vi "SyncTag_2.0 Test v2.vi"() -> ()   [LabVIEW 2017]
uses:
  <vilib>/Utility/error.llb/DialogType.ctl
  <vilib>/DAQmx/write.llb/DAQmx Write (Digital Wfm 1Chan NSamp).vi
  <vilib>/Waveform/DWDTOps.llb/DWDT Digital Size.vi
  <vilib>/DAQmx/create/channels.llb/DAQmx Create Channel (DO-Digital Output).vi
  <vilib>/DAQmx/configure/timing.llb/DAQmx Timing (Sample Clock).vi
  <vilib>/Waveform/DWDTOps.llb/DWDT Uncompress Digital.vi
  <vilib>/DAQmx/miscellaneous.llb/DAQmx Fill In Error Info.vi
  <resource>/objmgr/daqmx.rc
panel:
  in  "Sync Tagging":T1(tab)
  out "Minimum tagging period (pws)":u32=87
  out "Total tag data length (pws)":i32=86
  in  "TaggingPeriod (pws)":u32=155
  out "Tag data does NOT fit in period!!!":bool
  in  "Calculate recommended tag settings":bool
  in  "Validate tag settings":bool
  in  "Line(s)":tag="Dev1/port0/line0:7"
  out "Actual Sample Rate":dbl=1000.0 format="%0.2f"
  in  "Sample Clock Source":tag="PFI0"
  in  "Sample Rate":dbl=1000.0
  in  "TagMarkerDuration (pws)":i32=10
  out "digital waveform":digitalwaveform(graph)
  out "Tag num":u32=1
  in  "Min extra tag separation (pws)":u32=1
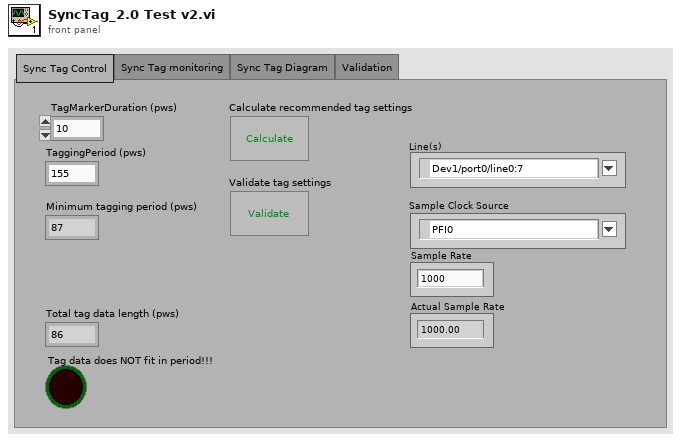
[diagram p1: front panel]
types:
  T1 = enum32{"Sync Tag Control", "Sync Tag monitoring", "Sync Tag Diagram", "Validation"}
  T2 = typedef "DialogType.ctl" = u16
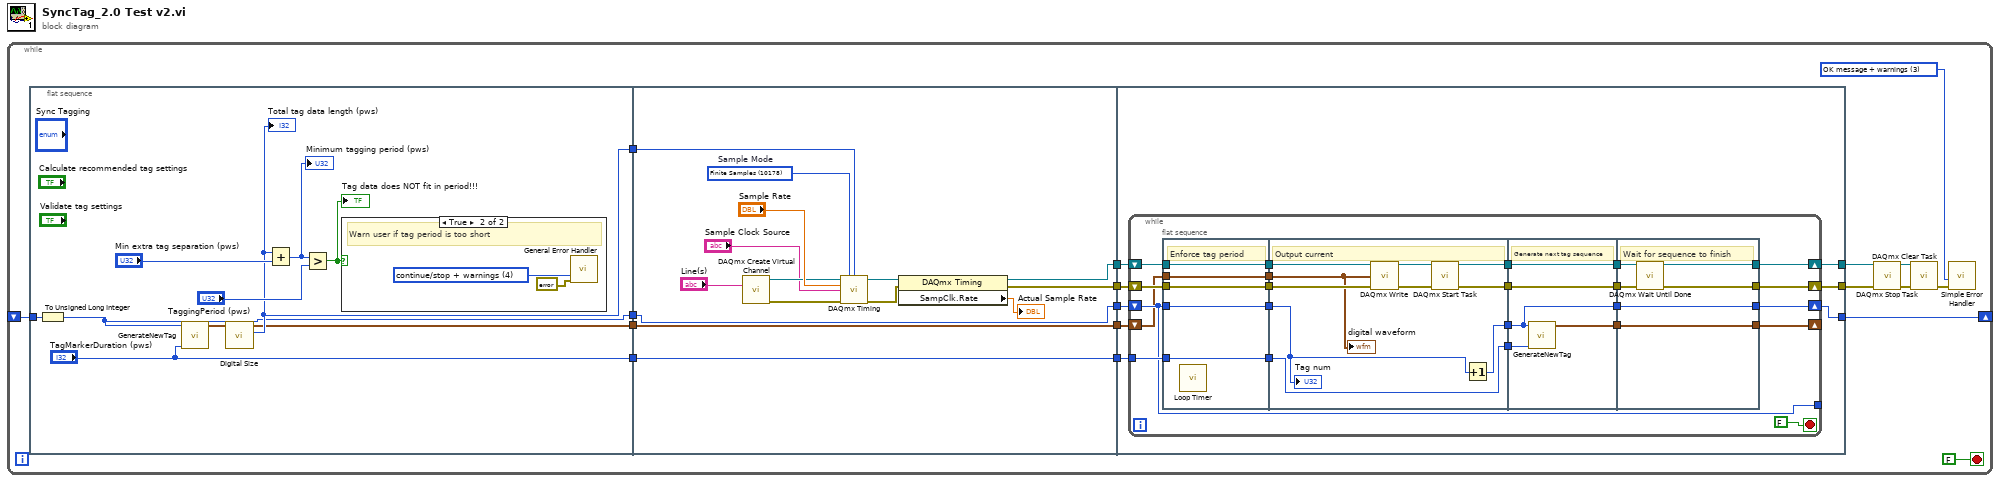
[diagram p0: block diagram]
diagram:
  n1 = while {
    shift-right: [w1] -> _
    shift-left: _ -> [w2]
    stop <- FALSE stop-if-true
    w6 = T2 3 items=["no dialog", "OK message", "continue or stop message", "OK message + warnings", "continue/stop + warnings"] ("type of dialog (OK msg:1)")
    n2 = flat-sequence {
      tunnel: ["TagMarkerDuration (pws)"] -> w18
      tunnel: [w22] -> w17
      tunnel: [w19] -> w16
      tunnel: [w21] -> w15
      tunnel: w2 -> [w20]
      tunnel: [w36] -> w14
      tunnel: [w35] -> w13
      tunnel: [w33] -> w12
      tunnel: w18 -> [w33]
      tunnel: w17 -> [w34]
      tunnel: [w32] -> w11
      tunnel: w16 -> [w32]
      tunnel: [w31] -> w10
      tunnel: w15 -> [w31]
      tunnel: [w53] -> w5
      tunnel: [w52] -> w4
      tunnel: w14 -> [w51]
      tunnel: w13 -> [w50]
      tunnel: w12 -> [w49]
      tunnel: w11 -> [w48]
      tunnel: w10 -> [w47]
      tunnel: [w46] -> w1
      frame #0 {
        n3 = To Unsigned Long Integer(number=w20) -> (unsigned 32bit integer=w19:u32)
        n4 = call "GenerateNewTag.vi"("TagMarkerDuration (pws)"="TagMarkerDuration (pws)", "Tag num"=w19) -> ("digital waveform"=w23:digitalwaveform)  [unwired: 9 in]
        n5 = call-poly <vilib>:"Digital Size.vi"("digital waveform in"=w23) -> ("number of samples"=w22:i32, "digital waveform out"=w21:digitalwaveform)  [unwired: 7 in, 2 out]
        "Total tag data length (pws)" <- w22
        n6 = Add(x=w22, y="Min extra tag separation (pws)") -> (x+y=w25:u32)
        "Minimum tagging period (pws)" <- w25
        n7 = Greater?(x=w25, y="TaggingPeriod (pws)") -> (0:w26:bool)
        "Tag data does NOT fit in period!!!" <- w26
        n8 = case shown="True" w26 {
          frame False {
          }
          frame True {
            w29 = T2 4 items=["no dialog", "OK message", "continue or stop message", "OK message + warnings", "continue/stop + warnings"] ("type of dialog (OK msg:1)")
            # "Warn user if tag period is too short"
            n9 = call <vilib>:"General Error Handler.vi"("type of dialog (OK msg:1)"=w29, "error in (no error)"=errorcluster {"status"=TRUE, "code"=-1967345148, "source"="Warning! Tag data does not fit in period. \nPlease increase tag period and restart VI."}) -> ()  [unwired: 9 in, 5 out]
          }
        }
      }
      frame #1 {
        w37 = 10178 items=["Finite Samples"=10178, "Continuous Samples"=10123, "Hardware Timed Single Point"=12522]  # Sample Mode
        n10 = call-poly <vilib>:"DAQmx Create Virtual Channel.vi"("lines"="Line(s)") -> ("task out"=w40:refnum<k21>, "error out"=w41:errorcluster)  [unwired: 13 in]
        n11 = call-poly <vilib>:"DAQmx Timing.vi"("task/channels in"=w40, "sample mode"=w37, "samples per channel"=w34, "rate"="Sample Rate", "source"="Sample Clock Source", "error in"=w41) -> ("task out"=w43:refnum<k21>, "error out"=w44:errorcluster)  [unwired: 8 in]
        n12 = property class="DAQmx Timing"(reference=w43, error in=w44) -> (reference out=w35:refnum<k21>, error out=w36:errorcluster, "SampClk.Rate"=→"Actual Sample Rate":dbl)
      }
      frame #2 {
        n13 = while {
          shift-right: [w74] -> w53
          shift-left: w50 -> [w76]
          shift-right: [w73] -> w52
          shift-left: w51 -> [w75]
          tunnel: w49 -> [w71]
          tunnel: [w70] -> _
          shift-right: [w69] -> w46
          shift-left: w48 -> [w70]
          shift-right: [w61] -> _
          shift-left: w47 -> [w64]
          stop <- FALSE ("stop") stop-if-true
          n14 = flat-sequence {
            tunnel: w70 -> [w78]
            tunnel: w71 -> [w79]
            tunnel: w75 -> [w80]
            tunnel: w76 -> [w81]
            tunnel: [w81] -> w68
            tunnel: [w80] -> w67
            tunnel: [w79] -> w66
            tunnel: [w78] -> w65
            tunnel: w64 -> [w77]
            tunnel: [w77] -> w62
            tunnel: w68 -> [w91]
            tunnel: w67 -> [w90]
            tunnel: w66 -> [w84]
            tunnel: w65 -> [w89]
            tunnel: [w88] -> w63
            tunnel: w62 -> [w85]
            tunnel: [w84] -> w60
            tunnel: [w83] -> w56
            tunnel: [w82] -> w54
            tunnel: w63 -> [w95]
            tunnel: w60 -> [w94]
            tunnel: [w95] -> w59
            tunnel: [w96] -> w58
            tunnel: [w93] -> w57
            tunnel: w56 -> [w93]
            tunnel: [w92] -> w55
            tunnel: w54 -> [w92]
            tunnel: [w101] -> w61
            tunnel: [w102] -> w69
            tunnel: [w97] -> w73
            tunnel: [w98] -> w74
            tunnel: w59 -> [w102]
            tunnel: w58 -> [w101]
            tunnel: w57 -> [w100]
            tunnel: w55 -> [w99]
            frame #0 {
              # "Enforce tag period"
              n15 = call "Loop Timer"() -> ()  [unwired: 1 in, 1 out]
            }
            frame #1 {
              # "Output current"
              n16 = call-poly <vilib>:"DAQmx Write.vi"("task/channels in"=w91, "data"=w85, "error in"=w90) -> ("task out"=w87:refnum<k21>, "error out"=w86:errorcluster)  [unwired: 10 in, 1 out]
              n17 = call <vilib>:"DAQmx Start Task.vi"("task/channels in"=w87, "error in"=w86) -> ("task out"=w83:refnum<k21>, "error out"=w82:errorcluster)  [unwired: 12 in]
              n18 = Increment(x=w89) -> (x+1=w88:u32)
              "digital waveform" <- w85
              "Tag num" <- w89
            }
            frame #2 {
              # "Generate next tag sequence"
              n19 = call "GenerateNewTag.vi"("TagMarkerDuration (pws)"=w94, "Tag num"=w95) -> ("digital waveform"=w96:digitalwaveform)  [unwired: 9 in]
            }
            frame #3 {
              # "Wait for sequence to finish"
              n20 = call <vilib>:"DAQmx Wait Until Done.vi"("task/channels in"=w100, "error in"=w99) -> ("task out"=w98:refnum<k21>, "error out"=w97:errorcluster)  [unwired: 12 in]
            }
          }
        }
      }
    }
    n21 = call <vilib>:"DAQmx Stop Task.vi"("task/channels in"=w5, "error in"=w4) -> ("task out"=w8:refnum<k21>, "error out"=w7:errorcluster)  [unwired: 12 in]
    n22 = call <vilib>:"DAQmx Clear Task.vi"("task in"=w8, "error in"=w7) -> ("error out"=w9:errorcluster)  [unwired: 13 in]
    n23 = call <vilib>:"Simple Error Handler.vi"("type of dialog (OK msg:1)"=w6, "error in (no error)"=w9) -> ()  [unwired: 3 in, 5 out]
  }
